vi "Dump OTP To File.vi"(8 "error in (no error)":errorcluster, 10 "filename":string, 11 "_hResourceContext":u32) -> (0 "error out":errorcluster, 2 "filename out":string, 3 "_hResourceContext out":u32)   [LabVIEW 2013, in "QCAWLAN_DLL.lvlib"]
doc: "QCA_DLL_Export void DumpOTPToFile(HANDLE _hResourceContext, char *filename);"
uses:
  QCAWLAN_DLL.lvlib
  QCAWLAN_DLL.dll
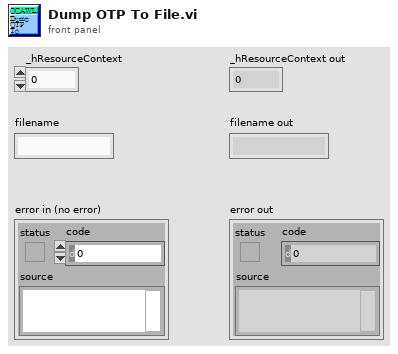
[diagram p1: front panel]
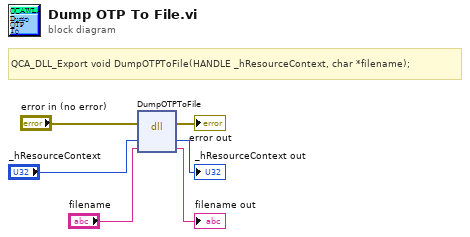
[diagram p0: block diagram]
diagram:
  # "QCA_DLL_Export void DumpOTPToFile(HANDLE _hResourceContext, char *filename);"
  n1 = dll-call lib="C:/Connectivity Client - MIMO/PlugIn/QCAWLAN_DLL.*" fn="DumpOTPToFile"(error in="error in (no error)", "_hResourceContext"="_hResourceContext", "filename"="filename") -> (error out=→"error out":errorcluster, "_hResourceContext"=→"_hResourceContext out":u32, "filename"=→"filename out":string)  [unwired: 3 in, 1 out]
